vi "flow-gen.io-compare.vi"(7 "Step Label":string, 9 "File":string, 10 "stepPointer (False Cond.)":string, 11 "Device Sensor Params":T2={"Input"="ain", "Comparison"=">=", "Setpoint"=0.0}) -> (3 "Step out":T3)   [LabVIEW 2024]
uses:
  controls/UiStepBuilder.ctl
  controls/type.step-builder.ctl
  controls/UiDeviceSensorParams.ctl
  controls/UiDeviceSensorEquality.ctl
panel:
  in  "Comparison":T1=">="
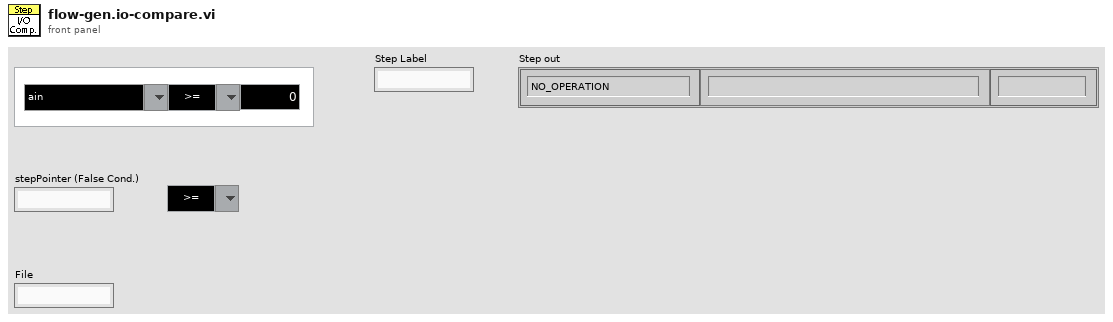
[diagram p1: front panel]
types:
  T1 = typedef "UiDeviceSensorEquality.ctl" = string
  T2 = typedef "UiDeviceSensorParams.ctl" = cluster{"Input":string, "Comparison":T1, "Setpoint":dbl}
  T3 = typedef "UiStepBuilder.ctl" = cluster{"Step Function":T4, "ParamString":string, "Step Label":string}
  T4 = typedef "type.step-builder.ctl" = enum16{"NO_OPERATION", "DELAY-JUMP", "DELAY", "JUMP", "COMPLETE", "SCHEDULER", "IRR-CHECK", "UNIT-CHECK", "UNIT-SAMPLE", "UNIT-DOSE", "LOG-REPORT", "LOG-MESSAGE", "IO-READ", "IO-READ-MANY", "IO-WRITE", "IO-COMPARE-OUT", "IO-COMPARE-IN", "PROC-START", "PROC-STOP", "PROC-LOAD", "PROC-IS-COMPLETED", "RECORD-MOVE", "GET-RH", "GET-UV", "GET-WD", "GET-WS", "OCS-CHECK", "OCS-RECORD"}
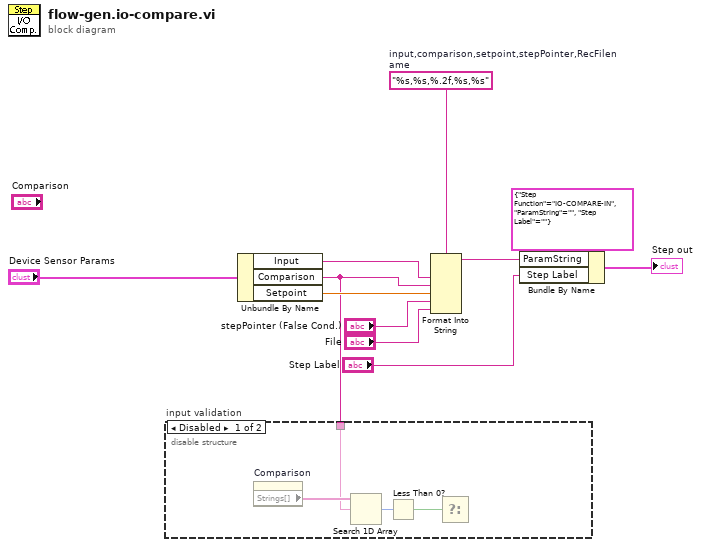
[diagram p0: block diagram]
diagram:
  w9 = "%s,%s,%.2f,%s,%s"  # input,comparison,setpoint,stepPointer,RecFilename
  n1 = Unbundle By Name("Device Sensor Params") -> ("Input"=w3:string, "Comparison"=w1:T1, "Setpoint"=w2:dbl)
  n2 = disable-structure "input validation" shown="Disabled" {
    disable-tunnel: w1 -> [w14 _]
    frame Disabled {
      n3 = property on="Comparison" class="CmbBox (strict)"() -> ("Strings[]"=w15:string[])  [unwired: 2 in, 2 out]
      n4 = Search 1D Array(1D array=w15, element=w14) -> (index of element=w13:i32)  [unwired: 1 in]
      n5 = Less Than 0?(x=w13) -> (x < 0?=w12:bool)
      n6 = Select(s=w12) -> ()  [unwired: 2 in, 1 out]
    }
    frame Enabled {
    }
  }
  n7 = Format Into String(format string=w9, w3, w1, w2, "stepPointer (False Cond.)", "File") -> (resulting string=w8:string)  [unwired: 2 in, 1 out]
  n8 = Bundle By Name(cluster=T3 {"Step Function"=enum."IO-COMPARE-IN", "ParamString"="", "Step Label"=""} ("FlowModeConstant 2"), "ParamString"=w8, "Step Label"="Step Label") -> (→"Step out":T3)
